vi "Update Templates Table for Spartan 5.0.vi"(8 "error in (no error)":errorcluster, 11 "Connection Refnum":T1) -> (0 "error out":errorcluster, 3 "Connection Refnum":T1)   [LabVIEW 2011]
uses:
  Summitek EXT/ODBC/SQL Controls/Connection Refnum.ctl
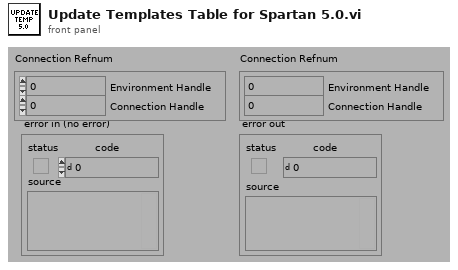
[diagram p1: front panel]
types:
  T1 = typedef "Connection Refnum.ctl" = cluster{"Environment Handle":i32, "Connection Handle":i32}
  T2 = typedef "Statement Refnum.ctl" = cluster{"Statement Handle":i32, "Parameter Number":u16}
  T3 = typedef "Field Record.ctl" = cluster{"ixField":i32, "iSequenceOrder":i32, "sxFieldId":string, "sxSequenceId":string, "sDisplayName":string, "sValue":string, "sUnits":string, "nDataType":T4, "nNextItem":T5, "fSystem":bool, "fSystemValue":bool, "fRequired":bool, "fSetAtTest":bool, "fTestField":bool, "fDeleted":bool, "fIndexed":bool, "fFreeList":bool}
  T4 = typedef "Field DataTypes.ctl" = enum32{"text", "numeric", "list", "timestamp", "boolean"}
  T5 = typedef "Field NextItem.ctl" = enum32{"Reset", "Retain", "Auto-Increment"}
  T6 = typedef "Template Record.ctl" = cluster{"ixTemplate":i32, "sxTemplateId":string, "sDescription":string, "sCreator":string, "tCreationDate":timestamp, "sModifier":string, "tModifiedDate":timestamp, "sType":string, "sStyle":string, "sFormat":string, "dWidth":dbl, "dHeight":dbl, "sFilename":string, "sScript":string, "sLayout":string, "sEditor":string, "sStyleProcess":string}
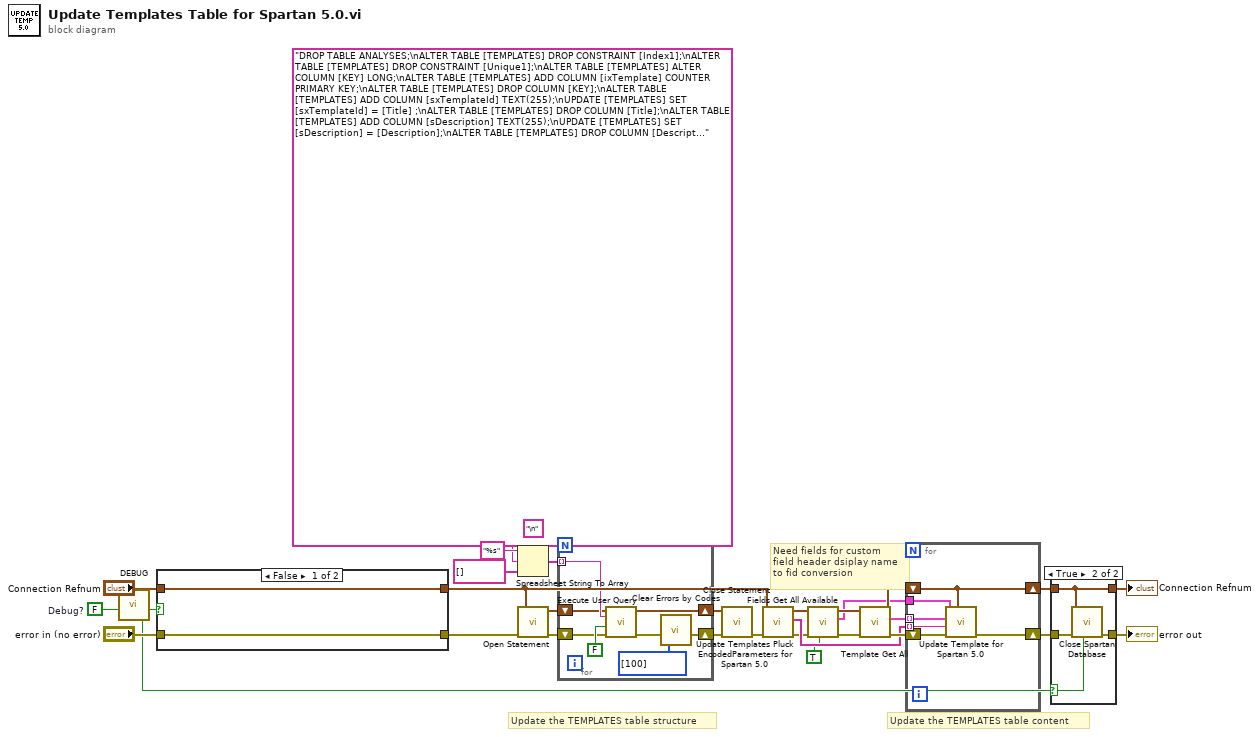
[diagram p0: block diagram]
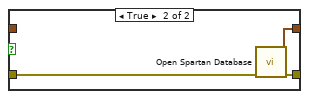
[diagram p2: hidden frame]
diagram:
  w16 = FALSE  # Debug?
  # "Update the TEMPLATES table content"
  # "Update the TEMPLATES table structure"
  # "Need fields for custom\nfield header dsiplay name\nto fid conversion"
  n1 = call "DEBUG.vi"("Dev DEBUG? (f)"=w16) -> ("DEBUG?"=w15:bool)  [unwired: 1 in, 5 out]
  n2 = case shown="False" w15 {
    tunnel: "Connection Refnum" -> [w32 _]
    tunnel: "error in (no error)" -> [w31 w35]
    tunnel: [w31 w34] -> w3
    tunnel: [w32 w33] -> w4
    frame False {
    }
    frame True {
      n3 = call "Open Spartan Database.vi"("error in (no error)"=w35) -> ("error out"=w34:errorcluster, "Connection Refnum"=w33:T1)  [unwired: 2 in, 7 out]
    }
  }
  n4 = Spreadsheet String To Array(delimiter (Tab)="\n", format string="%s", spreadsheet string="DROP TABLE ANALYSES;\nALTER TABLE [TEMPLATES] DROP CONSTRAINT [Index1];\nALTER TABLE [TEMPLATES] DROP CONSTRAINT [Unique1];\nALTER TABLE [TEMPLATES] ALTER COLUMN [KEY] LONG;\nALTER TABLE [TEMPLATES] ADD COLUMN [ixTemplate] COUNTER PRIMARY KEY;\nALTER TABLE [TEMPLATES] DROP COLUMN [KEY];\nALTER TABLE [TEMPLATES] ADD COLUMN [sxTemplateId] TEXT(255);\nUPDATE [TEMPLATES] SET [sxTemplateId] = [Title] ;\nALTER TABLE [TEMPLATES] DROP COLUMN [Title];\nALTER TABLE [TEMPLATES] ADD COLUMN [sDescription] TEXT(255);\nUPDATE [TEMPLATES] SET [sDescription] = [Description];\nALTER TABLE [TEMPLATES] DROP COLUMN [Description];\nALTER TABLE [TEMPLATES] ADD COLUMN [sCreator] TEXT(255);\nALTER TABLE [TEMPLATES] ADD COLUMN [tCreationDate] DATE;\nALTER TABLE [TEMPLATES] ADD COLUMN [sModifier] TEXT(255);\nALTER TABLE [TEMPLATES] ADD COLUMN [tModifiedDate] DATE;\nALTER TABLE [TEMPLATES] ADD COLUMN [sType] TEXT(255);\nUPDATE [TEMPLATES] SET [sType] = [Processing];\nALTER TABLE [TEMPLATES] DROP COLUMN [Processing];\nALTER TABLE [TEMPLATES] ADD COLUMN [sStyle] TEXT(255);\nALTER TABLE [TEMPLATES] ADD COLUMN [sStyleProcess] TEXT(255);\nUPDATE [TEMPLATES] SET [sStyle] = [Type];\nUPDATE [TEMPLATES] SET [sStyleProcess] = [Type];\nALTER TABLE [TEMPLATES] DROP COLUMN [Type];\nALTER TABLE [TEMPLATES] ADD COLUMN [sFormat] TEXT(255);\nALTER TABLE [TEMPLATES] ADD COLUMN [dWidth] FLOAT;\nALTER TABLE [TEMPLATES] ADD COLUMN [dHeight] FLOAT;\nALTER TABLE [TEMPLATES] ADD COLUMN [sFilename] TEXT(255);\nUPDATE [TEMPLATES] SET [sFilename] = [Path];\nALTER TABLE [TEMPLATES] DROP COLUMN [Path];\nALTER TABLE [TEMPLATES] ADD COLUMN [sScript] TEXT(255);\nALTER TABLE [TEMPLATES] ADD COLUMN [sLayout] TEXT(255);\nALTER TABLE [TEMPLATES] ADD COLUMN [sEditor] TEXT(255);" ("User Query"), array type (2D Dbl)=string[] []) -> (array=w29:string[])
  n5 = call "Open Statement.vi"("error in (no error)"=w3, "Connection Refnum"=w4) -> ("error out"=w26:errorcluster, "Statement Refnum"=w25:T2)  [unwired: 4 out]
  n6 = for {
    shift-right: [w36] -> w24
    shift-left: w26 -> [w40]
    tunnel: w29 -> [w42] mode=indexing
    shift-right: [w39] -> w23
    shift-left: w25 -> [w41]
    n7 = call "Execute User Query.vi"("error in (no error)"=w40, "Return Data? (f)"=FALSE, "User Query"=w42, "Statement Refnum"=w41) -> ("error out"=w37:errorcluster, "Statement Refnum"=w39:T2)  [unwired: 2 out]
    n8 = call "Clear Errors by Codes.vi"("Error Codes\nto Clear (Empty)"=i32[] [100] ("Error Codes\nto Clear (Empty)"), "error in (no error)"=w37) -> ("error out"=w36:errorcluster)  [unwired: 5 out]
  }
  n9 = call "Close Statement.vi"("error in (no error)"=w24, "Statement Refnum"=w23) -> ("error out"=w14:errorcluster)  [unwired: 5 out]
  n10 = call "Update Templates Pluck EncodedParameters for Spartan 5.0.vi"("error in (no error)"=w14, "Connection Refnum"=w4) -> ("error out"=w8:errorcluster, "EncodedParameters"=w10:string[], "Connection Refnum"=w7:T1)  [unwired: 7 out]
  n11 = call "Fields Get All Available.vi"("Combine All? (f)"=TRUE, "error in (no error)"=w8, "Connection Refnum"=w7) -> ("error out"=w5:errorcluster, "System or ALL Combined Fields"=w1:T3[], "Connection Refnum"=w6:T1)  [unwired: 2 in, 4 out]
  n12 = call "Template Get All.vi"("error in (no error)"=w5, "Connection Refnum"=w6) -> ("error out"=w12:errorcluster, "Templates"=w11:T6[], "Connection Refnum"=w13:T1)  [unwired: 1 in, 6 out]
  n13 = for {
    shift-right: [w44] -> w22
    shift-left: w12 -> [w49]
    shift-right: [w45] -> w21
    shift-left: w13 -> [w45]
    tunnel: w11 -> [w48] mode=indexing
    tunnel: w10 -> [w47] mode=indexing
    tunnel: w1 -> [w46]
    n14 = call "Update Template for Spartan 5.0.vi"("Connection Refnum"=w45, "error in (no error)"=w49, "EncodedParameters"=w47, "Old Template Record"=w48, "All Fields"=w46) -> ("error out"=w44:errorcluster)  [unwired: 6 out]
  }
  n15 = case shown="True" w15 {
    selector: w15 -> [_ w53]
    tunnel: w22 -> [w51 w55]
    tunnel: w21 -> [w50 w52]
    tunnel: [w50 w52] -> w20
    tunnel: [w51 w54] -> w19
    frame False {
    }
    frame True {
      n16 = call "Close Spartan Database.vi"("Force Close? (f)"=w53, "error in (no error)"=w55, "Connection Refnum"=w52) -> ("error out"=w54:errorcluster)  [unwired: 2 in, 6 out]
    }
  }
  "error out" <- w19
  "Connection Refnum" <- w20
